vi "CSM - Broadcast Status Change.vi"(0 "Status With Arguments":string, 5 "State Queue":string, 7 "Broadcast? (T)":bool=TRUE) -> (6 "Remaining States":string)   [LabVIEW 2017, in "Communicable State Machine.lvlib"]
doc: "Broadcasts a status change to the system. CSM modules with registered states will receive this status change. For example:\n\n // Broadcast status change\n Status >> Arguments -><broadcast>\n\n> [!NOTE]\n> <b>CSM State Queue Operation API</b>\n>\n> This type of API only concatenates message strings and does not send messages directly. The message is sent and the operation executed within the Parse State Queue++ VI. Unlike the Message Building API, this type of API includes a CSM state queue string input, which is equivalent to inserting a message into the state queue.\n\n-- <b>Controls</b> --\n- <b>Status with Arguments</b>: The status and arguments to be broadcast. This input supports multiple lines and each state line will have `-><broadcast>` appended.\n- <b>State Queue</b>: The entire state queue is connected to this input.\n- <b>Broadcast? (T)</b>: Specifies whether to broadcast.\n\n-- <b>Indicators</b> --\n- <b>Remaining States</b>: Returns all concatenated states and arguments."
uses:
  Communicable State Machine.lvlib
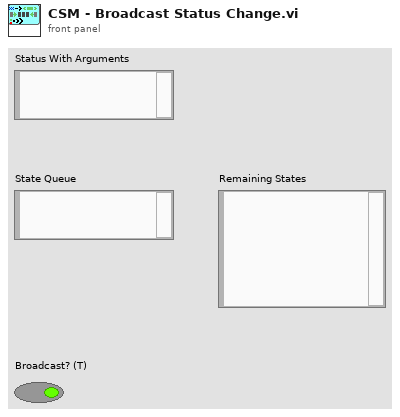
[diagram p1: front panel]
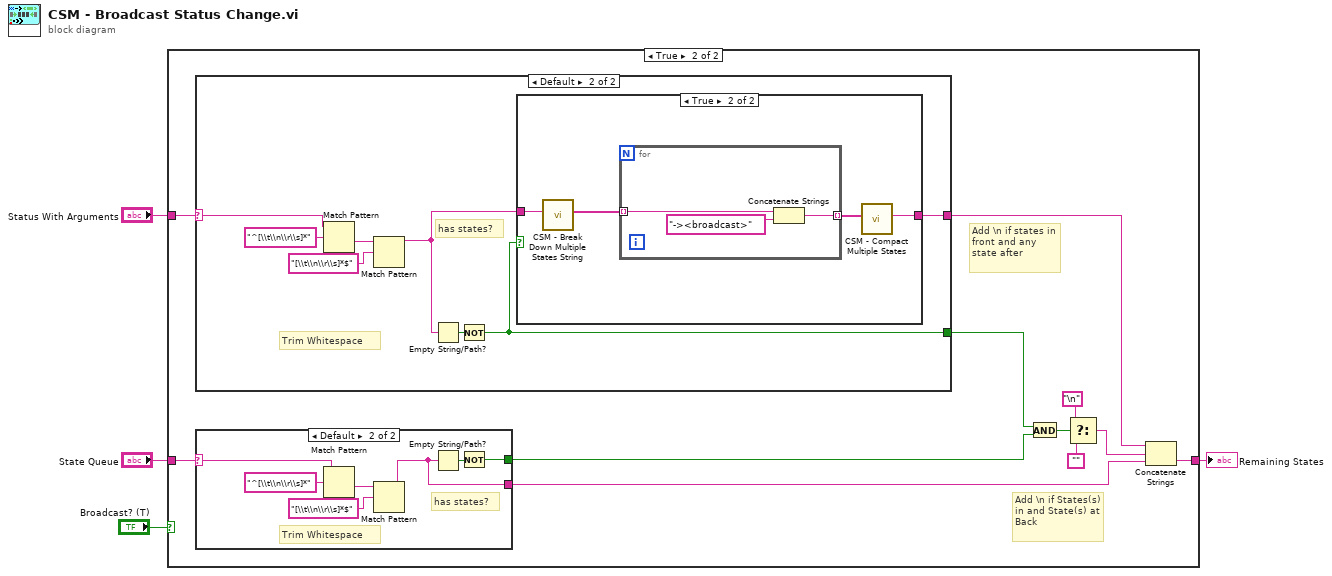
[diagram p0: block diagram]
diagram:
  n1 = case shown="True" "Broadcast? (T)" {
    tunnel: [w5 w16] -> w4
    tunnel: "Status With Arguments" -> [_ w8]
    tunnel: "State Queue" -> [w5 w7]
    frame False {
    }
    frame True {
      # "Add \\n if States(s) in and State(s) at Back"
      # "Add \\n if states in front and any state after"
      n2 = case shown="Default" w8 {
        selector: w8 -> [_ w27]
        tunnel: [_ w24] -> w15
        tunnel: [_ w25] -> w10
        frame "" {
        }
        frame Default {
          # "Trim Whitespace"
          # "has states?"
          n3 = Match Pattern(string=w27, regular expression="^[\\t\\n\\r\\s]*") -> (after substring=w29:string)  [unwired: 1 in, 3 out]
          n4 = Match Pattern(string=w29, regular expression="[\\t\\n\\r\\s]*$") -> (before substring=w26:string)  [unwired: 1 in, 3 out]
          n5 = Empty String/Path?(string/path=w26) -> (empty?=w31:bool)
          n6 = Not(x=w31) -> (.not. x?=w24:bool)
          n7 = case shown="True" w24 {
            tunnel: w26 -> [w32 w36]
            tunnel: [w32 w33] -> w25
            frame False {
            }
            frame True {
              n8 = call "CSM - Break Down Multiple States String.vi"("States"=w36) -> ("Multiple States"=w35:string[])  [unwired: 10 in]
              n9 = for {
                tunnel: [w39] -> w34 mode=indexing
                tunnel: w35 -> [w37] mode=indexing
                n10 = Concatenate Strings(w37, "-><broadcast>" ("string")) -> (w39:string)
              }
              n11 = call "CSM - Compact Multiple States.vi"("Multiple States"=w34) -> ("States"=w33:string)  [unwired: 9 in]
            }
          }
        }
      }
      n12 = case shown="Default" w7 {
        selector: w7 -> [_ w17]
        tunnel: [_ w22] -> w6
        tunnel: [_ w18] -> w9
        frame "" {
        }
        frame Default {
          # "Trim Whitespace"
          # "has states?"
          n13 = Match Pattern(string=w17, regular expression="^[\\t\\n\\r\\s]*") -> (after substring=w20:string)  [unwired: 1 in, 3 out]
          n14 = Match Pattern(string=w20, regular expression="[\\t\\n\\r\\s]*$") -> (before substring=w18:string)  [unwired: 1 in, 3 out]
          n15 = Empty String/Path?(string/path=w18) -> (empty?=w23:bool)
          n16 = Not(x=w23) -> (.not. x?=w22:bool)
        }
      }
      n17 = And(x=w15, y=w6) -> (x .and. y?=w14:bool)
      n18 = Select(t="\n", s=w14, f="") -> (s? t:f=w13:string)
      n19 = Concatenate Strings(w10, w13, w9) -> (w16:string)
    }
  }
  "Remaining States" <- w4
